vi "Inner_Port_Offset.vi"() -> ()   [LabVIEW 2019]
uses:
  ArgosLib/ArgosLib.lvlib
panel:
  in  "Port in range?":bool
  out "K":dbl
  out "A":dbl
  out "G":dbl
  out "X":dbl
  out "B":dbl
  out "T":dbl
  in  "D":dbl
  in  "Theta":dbl
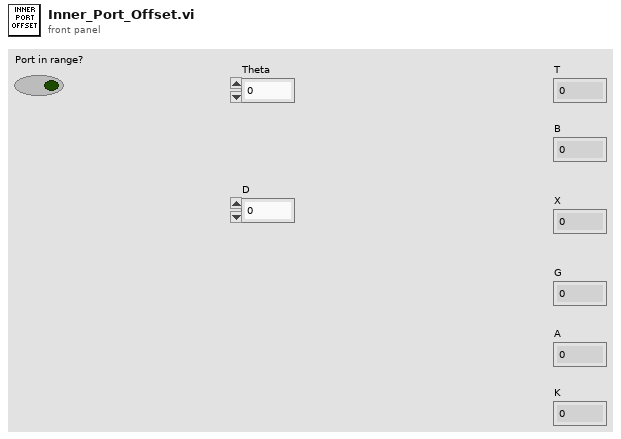
[diagram p1: front panel]
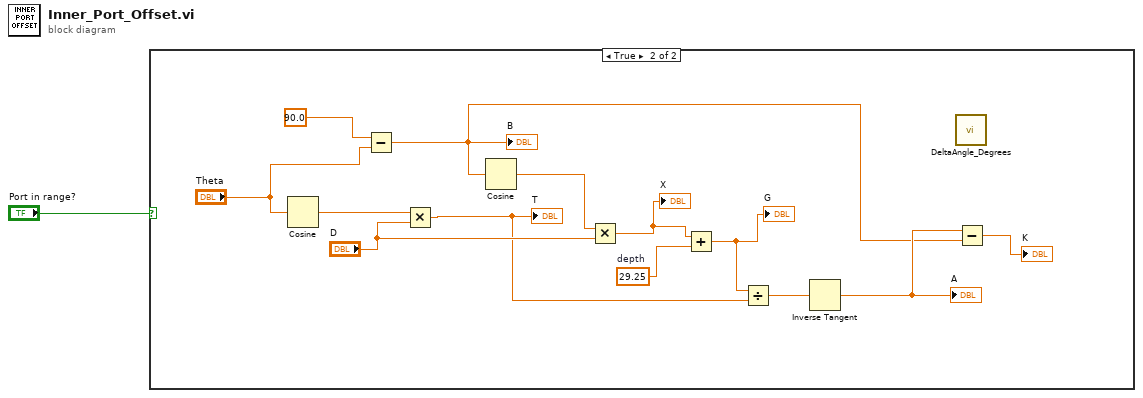
[diagram p0: block diagram]
diagram:
  n1 = case shown="True" "Port in range?" {
    frame False {
    }
    frame True {
      w8 = 29.25  # depth
      n2 = Cosine(x="Theta") -> (cos(x)=w13:dbl)
      n3 = Subtract(x=90.0, y="Theta") -> (x-y=w3:dbl)
      "B" <- w3
      n4 = Multiply(x=w13, y="D") -> (x*y=w6:dbl)
      "T" <- w6
      n5 = Cosine(x=w3) -> (cos(x)=w10:dbl)
      n6 = Multiply(x=w10, y="D") -> (x*y=w9:dbl)
      "X" <- w9
      n7 = Add(x=w9, y=w8) -> (x+y=w7:dbl)
      "G" <- w7
      n8 = Divide(x=w7, y=w6) -> (x/y=w5:dbl)
      n9 = Inverse Tangent(1:w5) -> (0:w4:dbl)
      "A" <- w4
      n10 = call "DeltaAngle_Degrees.vi"() -> ()  [unwired: 2 in, 1 out]
      n11 = Subtract(x=w4, y=w3) -> (x-y=→"K":dbl)
    }
  }
